vi "Get All Outgoing Ports.vi"(8 "error in":errorcluster, 11 "Ballard ARINC 429 ref":T1=18446744073709551615 format="%.0x") -> (0 "error out":errorcluster, 2 "Port refs":T1[](array[typedef]) format="%.0x", 3 "Ballard ARINC 429 ref out":T1 format="%.0x")   [LabVIEW 2020, in "Ballard ARINC 429 Scripting.lvlib"]
uses:
  Ballard ARINC 429 Scripting.lvlib
  Constants.vi
  <vilib>/NI VeriStand/Custom Device Tools/Custom Device Utility Library/Custom Device Utility Library.lvlib
  <vilib>/NI VeriStand/Custom Device Tools/Custom Device Utility Library/NI VeriStand - Search for Item by GUID.vi
  <vilib>/NI VeriStand/Custom Device Tools/Custom Device Utility Library/NI VeriStand - Search for All Items by GUID.vi
  <vilib>/NI VeriStand/Custom Device API/Custom Device Item Ref.ctl
  <vilib>/NI VeriStand/Custom Device API/Custom Device API.lvlib
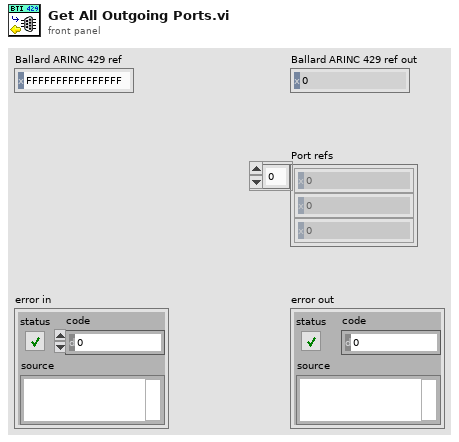
[diagram p1: front panel]
types:
  T1 = typedef "Custom Device API.lvlib/Custom Device Item Ref.ctl" = u64
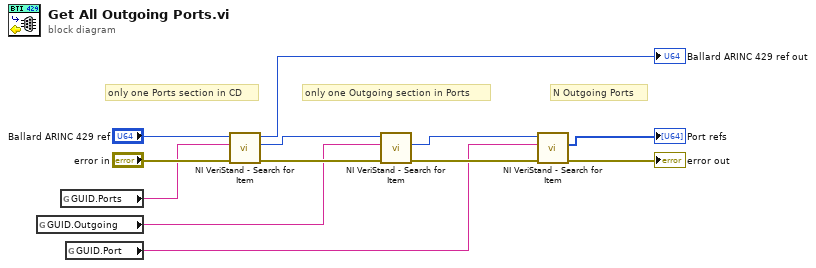
[diagram p0: block diagram]
diagram:
  # "N Outgoing Ports"
  # "only one Outgoing section in Ports"
  # "only one Ports section in CD"
  n1 = global read "Constants.vi" "GUID.Outgoing"() -> (w8:string)
  n2 = global read "Constants.vi" "GUID.Ports"() -> (w7:string)
  n3 = global read "Constants.vi" "GUID.Port"() -> (w5:string)
  n4 = call-poly <vilib>:"NI VeriStand - Search for Item.vi"("error in"="error in", "Item GUID"=w7, "Section Ref in"="Ballard ARINC 429 ref") -> ("error out"=w10:errorcluster, "Item Ref"=w9:T1, "Section Ref out"=→"Ballard ARINC 429 ref out":T1)  [unwired: 5 in, 1 out]
  n5 = call-poly <vilib>:"NI VeriStand - Search for Item.vi"("error in"=w10, "Item GUID"=w8, "Section Ref in"=w9) -> ("error out"=w6:errorcluster, "Item Ref"=w4:T1)  [unwired: 5 in, 2 out]
  n6 = call-poly <vilib>:"NI VeriStand - Search for Item.vi"("error in"=w6, "Item GUID"=w5, "Section Ref in"=w4) -> ("error out"=→"error out":errorcluster, "Item Refs"=→"Port refs":T1[])  [unwired: 5 in, 2 out]
